vi "Select Log Data.vi"(9 "Log Active":bool[][](array[boolean]), 10 "Scaled":sgl[](array[numeric]), 11 "Raw":sgl[](array[numeric])) -> (2 "Raw Out":string[](array[string]), 3 "Scaled Out":string[](array[string]))   [LabVIEW 2018]
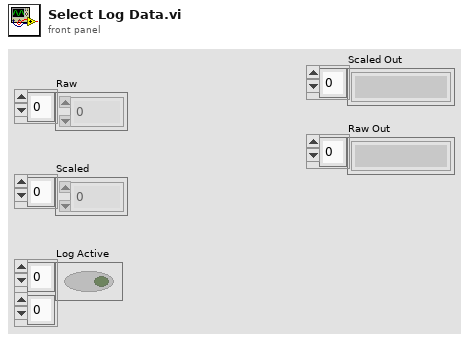
[diagram p1: front panel]
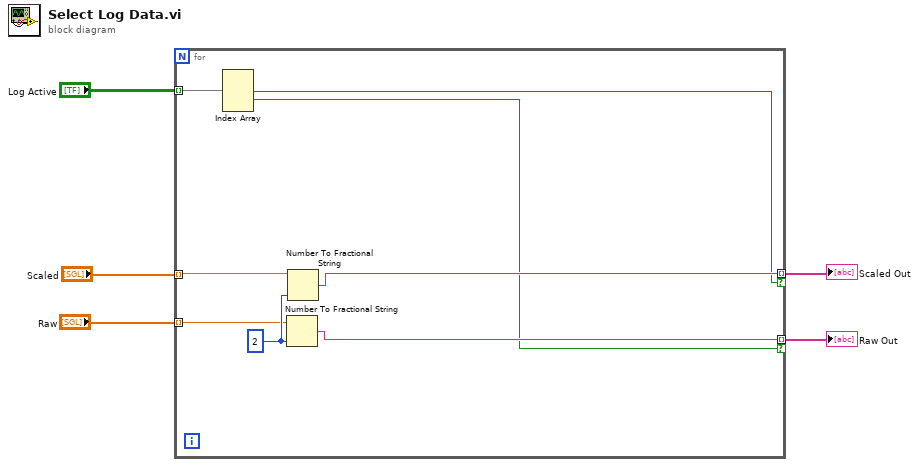
[diagram p0: block diagram]
diagram:
  n1 = for {
    tunnel: "Scaled" -> [w12] mode=indexing
    tunnel: "Raw" -> [w8] mode=indexing
    tunnel: "Log Active" -> [w13] mode=indexing
    tunnel: [w10] -> w2 mode=indexing if=w7
    tunnel: [w9] -> w1 mode=indexing if=w6
    w11 = i16 2 ("precision (6)")
    n2 = Index Array(array=w13) -> (element #1=w7:bool, element #2=w6:bool)  [unwired: 3 in, 1 out]
    n3 = Number To Fractional String(number=w8, precision (6)=w11) -> (F-format string=w9:string)  [unwired: 2 in]
    n4 = Number To Fractional String(number=w12, precision (6)=w11) -> (F-format string=w10:string)  [unwired: 2 in]
  }
  "Scaled Out" <- w2
  "Raw Out" <- w1
